vi "ingest.trigger.vi"(6 "Properties and Labels":T1, 7 "Timestamp Metadata":refnum<class "timestampMetadata.lvclass">, 8 "error in":errorcluster, 9 "Title and Description":cluster{"Title":string, "Description":string}, 10 "S3 Path to File":string, 11 "Nominal Client in":refnum<class "Nominal Client.lvclass">) -> (0 "error out":errorcluster, 1 "Information":T2, 2 "datasetRid":string, 3 "Nominal Client out":refnum<class "Nominal Client.lvclass">, 4 "Response":string)   [LabVIEW 2020, in "Nominal Client.lvclass"]
doc: "<b> DEPRECIATED METHOD: Use Ingest All.vi for new projects </b>\n\nTriggers an ingest job for the given data source. The ingest job will be processed asynchronously.\n\nTo set the timestamp metadata, use the Timestamp Metadata Create function."
uses:
  Nominal Client.lvclass
  timestampMetadata/timestampMetadata.lvclass
  Nominal Client.lvclass/Nominal Client.ctl
  nominal types/workspace/workspace.lvclass/workspace.ctl
  4b965f09-dc68-4d5e-a5c1-32d476accfd4.vi
  3b653ec0-b3f4-4e20-9ef1-15560b52d02f.vi
  dc60078f-5e64-4343-b872-0272d4308f69.vi
  trace.payload_received.vi
  error.vi
  trace.payload_sent.vi
  create.authorization_header.vi
  workspace.get.vi
  <vilib>/JDP Science/JSONtext/Merge into Object.vi
  workspace.add_to_payload.vi/88650e10-de3e-481c-85db-71cb0fdf4485.vi
  nominal types/workspace/rid.get.vi
  trace.calling_method.vi
  error.vi/859f8e04-e495-489b-b5b4-7ac163f56130.vi
  <vilib>/JDP Science/JDP Science Common Utilities/Trim Whitespace__JDP.vi
  <vilib>/AdvancedString/1D String Array to Delimited String.vi
  api_token.get.vi
  <vilib>/JDP Science/JSONtext/Variant to JSON Text.vi
  <vilib>/JDP Science/JSONtext/Array of Variants to JSON Object.vi
  <vilib>/JDP Science/JSONtext/Set Item.vi
  <vilib>/JDP Science/JSONtext/Get all Object Items.vi
  <vilib>/JDP Science/JSONtext/Set Multiple Object Items.vi
  <vilib>/Utility/libraryn.llb/Get File Extension.vi
  log_file.write.vi
  submodules/reqwest-labview/lv-src/reqwest/post.vi
  <vilib>/Utility/error.llb/Error Cluster From Error Code.vi
  <vilib>/JDP Science/JSONtext/JSON text to Variant.vi
  <vilib>/JDP Science/JSONtext/LVClass Serializer/JSONtext LVClass Serializer.lvclass
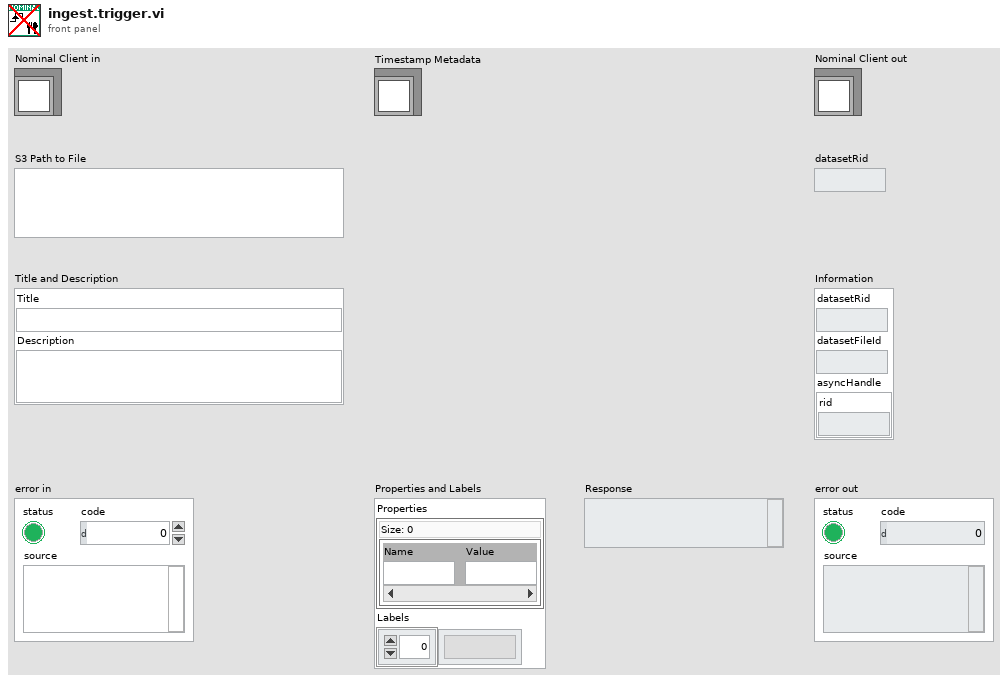
[diagram p1: front panel]
types:
  T1 = cluster{"Properties":map{string, string}, "Labels":string[]}
  T2 = cluster{"datasetRid":string, "datasetFileId":string, "asyncHandle":cluster{"rid":string}}
  T3 = cluster{"type":string, "s3":cluster{"path":string}}
  T4 = cluster{"source":cluster{"type":string, "s3":cluster{"path":string}}, "properties":string, "labels":string[], "datasetName":string, "datasetDescription":string}
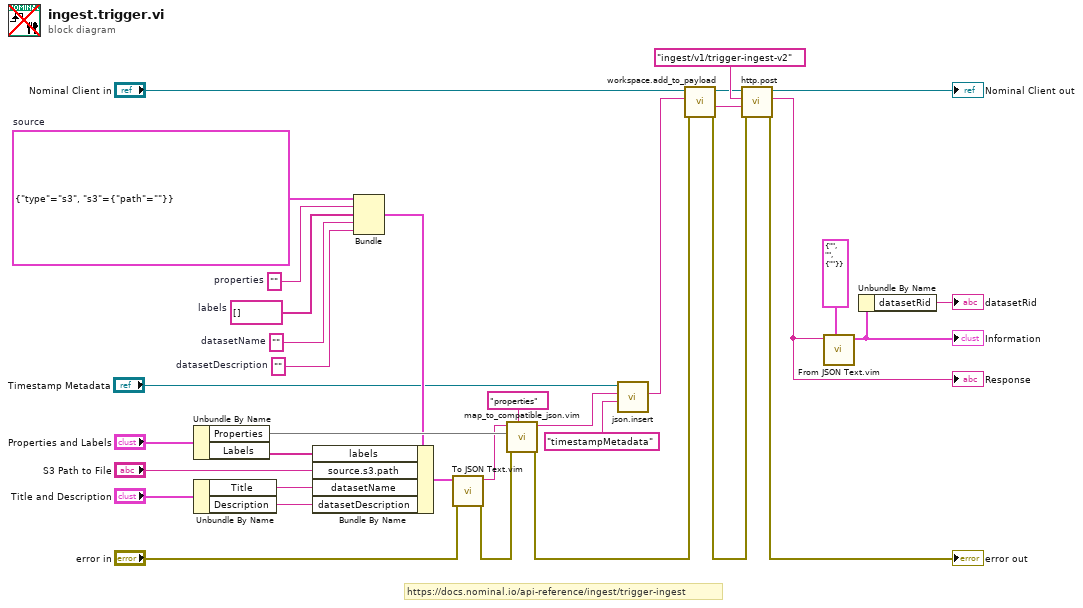
[diagram p0: block diagram]
diagram:
  w26 = ""  # datasetDescription
  w27 = ""  # datasetName
  w29 = ""  # properties
  w28 = string[] []  # labels
  w31 = T3 {"type"="s3", "s3"={"path"=""}}  # source
  # "https://docs.nominal.io/api-reference/ingest/trigger-ingest"
  n1 = Unbundle By Name("Properties and Labels") -> ("Properties"=w19:map{string, string}, "Labels"=w20:string[])
  n2 = Unbundle By Name("Title and Description") -> ("Title"=w22:string, "Description"=w23:string)
  n3 = Bundle("source"=w31, "properties"=w29, "labels"=w28, "datasetName"=w27, "datasetDescription"=w26) -> (w14:T4)  [unwired: 1 in]
  n4 = Bundle By Name(cluster=w14, "labels"=w20, "source.s3.path"="S3 Path to File", "datasetName"=w22, "datasetDescription"=w23) -> (w12:T4)
  n5 = call "To JSON Text.vim"("error in (no error)"="error in", "Anything"=w12) -> ("error out"=w10:errorcluster, "<JSON>"=w11:string)  [unwired: 8 in]
  n6 = call "map_to_compatible_json.vim"("JSON Path"="properties" ("Data Name"), "error in"=w10, "Map"=w19, "JSON in"=w11) -> ("error out"=w2:errorcluster, "JSON out"=w8:string)  [unwired: 6 in]
  n7 = call "json.insert.vi"("Object Name"="timestampMetadata", "JSON in"=w8, "timestampMetadata in"="Timestamp Metadata") -> ("JSON out"=w4:string)  [unwired: 6 in, 2 out]
  n8 = call "workspace.add_to_payload.vi"("error in"=w2, "JSON payload in"=w4, "Nominal Client in"="Nominal Client in") -> ("error out"=w1:errorcluster, "JSON payload out"=w3:string, "Nominal Client out"=w5:refnum<class "Nominal Client.lvclass">)  [unwired: 6 in]
  n9 = call "http.post.vi"("error in"=w1, "Request body"=w3, "Path"="ingest/v1/trigger-ingest-v2", "Nominal Client in"=w5) -> ("error out"=→"error out":errorcluster, "Response"=w15:string, "Nominal Client out"=→"Nominal Client out":refnum<class "Nominal Client.lvclass">)  [unwired: 5 in]
  "Response" <- w15
  n10 = call "From JSON Text.vim"("Data Type and Default Value"=T2 {"datasetRid"="", "datasetFileId"="", "asyncHandle"={"rid"=""}} ("Information"), "JSON"=w15) -> ("Data out"=w17:T2)  [unwired: 8 in, 1 out]
  "Information" <- w17
  n11 = Unbundle By Name(w17) -> ("datasetRid"=→"datasetRid":string)
